vi "input processing.vi"(11 "String":string) -> (2 "inputan 5":bool, 3 "substring before match":string)   [LabVIEW 2017]
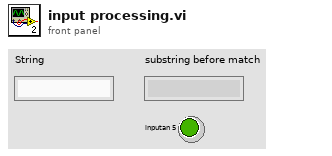
[diagram p1: front panel]
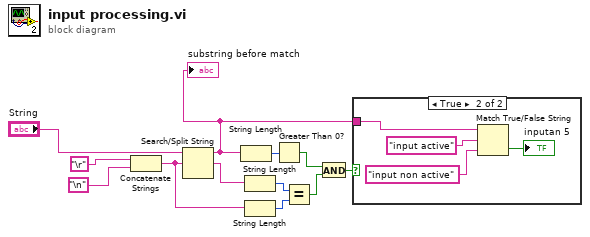
[diagram p0: block diagram]
diagram:
  n1 = Concatenate Strings("\r", "\n") -> (w5:string)
  n2 = Search/Split String(string="String", search string/char (-)=w5) -> (substring before match=w12:string, match + rest of string=w6:string)  [unwired: 1 in, 1 out]
  "substring before match" <- w12
  n3 = String Length(string=w12) -> (length=w4:i32)
  n4 = String Length(string=w6) -> (length=w8:i32)
  n5 = String Length(string=w5) -> (length=w7:i32)
  n6 = Greater Than 0?(x=w4) -> (x > 0?=w10:bool)
  n7 = Equal?(x=w8, y=w7) -> (x = y?=w9:bool)
  n8 = And(x=w10, y=w9) -> (x .and. y?=w11:bool)
  n9 = case shown="True" w11 {
    tunnel: w12 -> [_ w15]
    frame False {
    }
    frame True {
      n10 = Match True/False String(2:"input non active" ("false string"), 3:"input active", 4:w15) -> (0:→"inputan 5":bool)  [unwired: 1 out]
    }
  }
